vi "20220105_ArbitraryWaveGen.vi"() -> ()   [LabVIEW 2021]
doc: "This VI demonstrates the use of the Arbitrary Wave signal generator VI. The top waveform graph shows the arbitrary wave array generated using the input controls. The diagram shows how to convert from these common frequency units to the \"normalized\" frequency units of cycles/sample (cycles/sample is the unit used by the Sine Wave, Triangle Wave, Square Wave, Sawtooth Wave, Arbitrary Wave, and Chirp Pattern VIs.) The Waveform Pattern simply plots the points given in the input array Wave Table, which represents 1 cycle of the arbitrary wave. If reset phase is set to OFF (false), the Arbitrary Wave VI will output the next samples of the waveform, preserving a continuously smooth phase."
uses:
  <vilib>/Utility/file.llb/Read Delimited Spreadsheet (DBL).vi
  <vilib>/Analysis/NI_AALBase.lvlib
panel:
  out "Column 1":dbl[](graph)
  out "Column 2":dbl[](graph)
  in  "Frequency Unit":u16(ring) items=["Hz", "cycles"]
  in  "Stop":bool
  in  "Reset phase":bool
  in  "Sampling rate (Hz)":dbl=100.0 step=1.0 format="%#.3g"
  out "Waveform Pattern":dbl[](graph)
  in  "interpolation":i32(ring)=1 items=["none", "linear"]
  in  "Frequency":dbl=2.01 step=1.0 format="%0.2f"
  in  "Amplitude":dbl(slide)=3.7755102040816326 scale=0.0..5.0
  # "Overview: Demonstrates the use of the Arbitrary Wave VI.\nRequirements: LabVIEW Full Development System\nInstructions: \n1. Run the VI.\n2. Adjust the Frequency and interpolation method.  \n3. Edit a single cycle of the arbitrary waveform by changing the Wave Table array, plotted in the Waveform Pattern graph. \n4. Click Stop to stop the VI."
  # "Signal Generation Parameters"
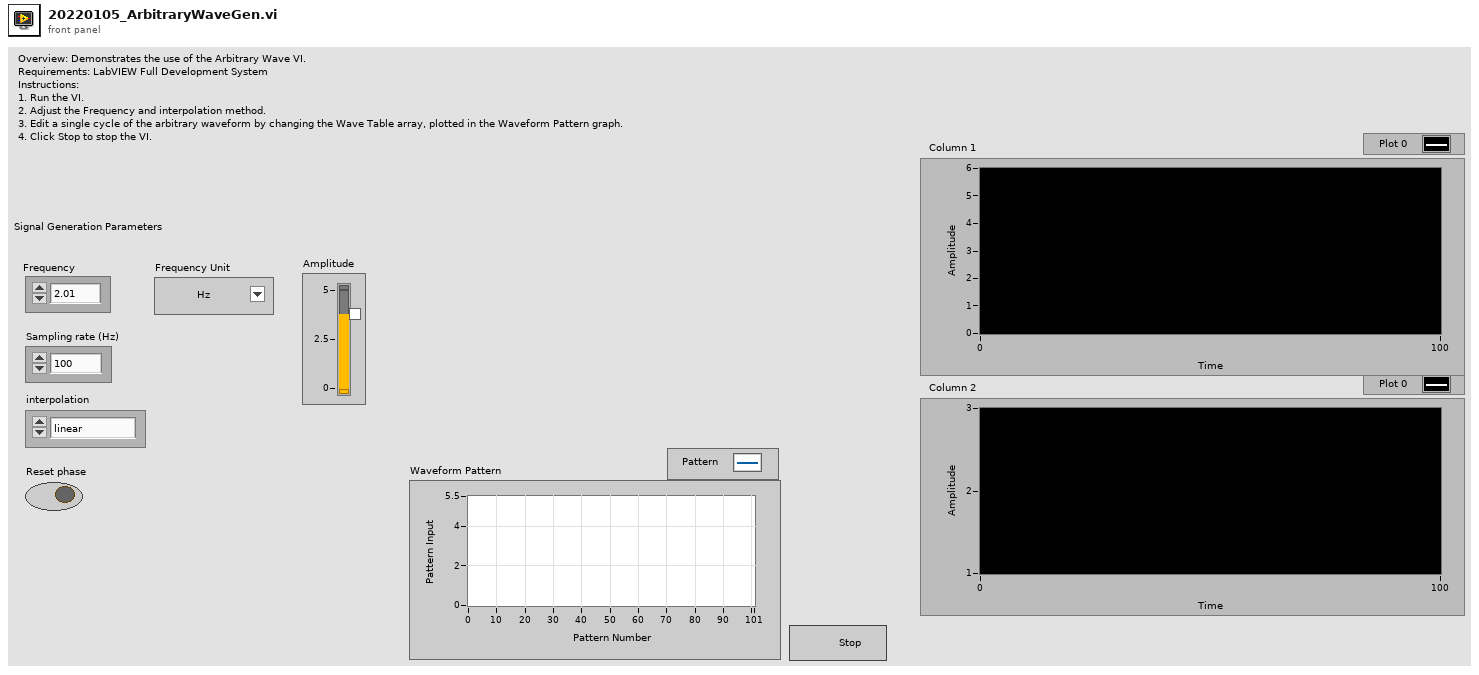
[diagram p1: front panel]
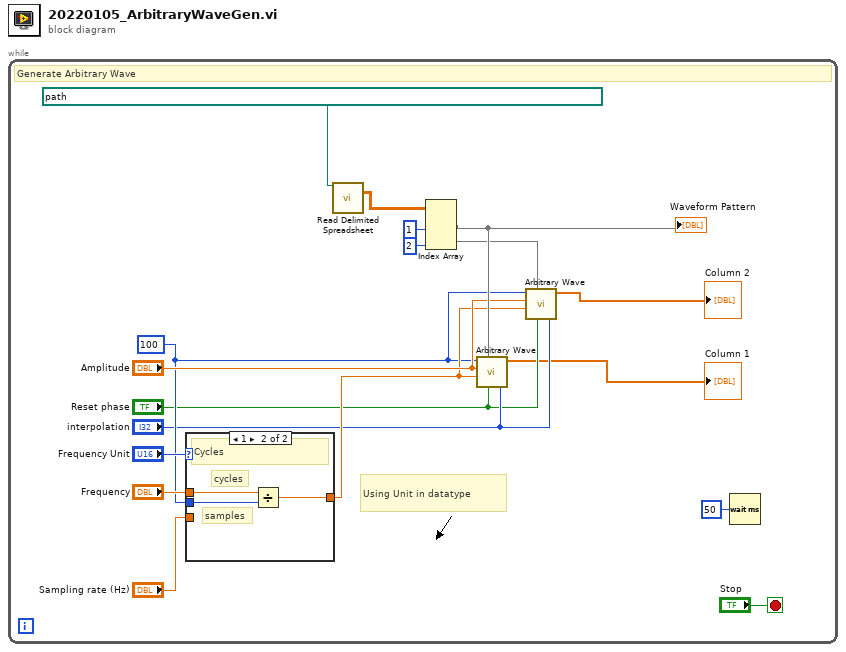
[diagram p0: block diagram]
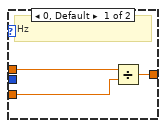
[diagram p2: hidden frame]
diagram:
  n1 = while {
    stop <- "Stop" stop-if-true
    w5 = 100 ("samples")
    # "Using Unit in datatype"
    # "Generate Arbitrary Wave"
    n2 = case shown="1" "Frequency Unit" {
      tunnel: [w21 w23] -> w6
      tunnel: w5 -> [_ w24]
      tunnel: "Frequency" -> [w20 w22]
      tunnel: "Sampling rate (Hz)" -> [w19 _]
      frame 0, Default {
        # "Hz"
        n3 = Divide(x=w20, y=w19) -> (x/y=w21:dbl)
      }
      frame 1 {
        # "samples"
        # "cycles"
        # "Cycles"
        n4 = Divide(x=w22, y=w24) -> (x/y=w23:dbl)
      }
    }
    n5 = call-poly <vilib>:"Read Delimited Spreadsheet.vi"("file path (dialog if empty)"=path "C:/Users/joe.kao/OneDrive - eCloudvalley Digital Technology/桌面/nPM1100_WaveformTable.txt") -> ("all rows"=w12:dbl[][])  [unwired: 9 in, 5 out]
    n6 = Index Array(array=w12, index (col) #1=1 ("disabled index (col)"), index (col) #2=2 ("index (col)")) -> (element #1=w10:dbl[], element #2=w8:dbl[])  [unwired: 2 in]
    "Waveform Pattern" <- w10
    n7 = call <vilib>:"Arbitrary Wave.vi"("interpolation"="interpolation", "reset phase"="Reset phase", "Wave Table"=w10, "frequency"=w6, "amplitude"="Amplitude", "samples"=w5) -> ("arbitrary wave"=→"Column 1":dbl[])  [unwired: 1 in, 2 out]
    n8 = call <vilib>:"Arbitrary Wave.vi"("interpolation"="interpolation", "reset phase"="Reset phase", "Wave Table"=w8, "frequency"=w6, "amplitude"="Amplitude", "samples"=w5) -> ("arbitrary wave"=→"Column 2":dbl[])  [unwired: 1 in, 2 out]
    n9 = Wait (ms)(milliseconds to wait=u32 50) -> ()  [unwired: 1 out]
  }
